vi "Write Switch Setting.vi"(8 "error in (no error)":errorcluster, 10 "Switch Setting":T1, 11 "Switch configuration":refnum<class "Switch configuration.lvclass">) -> (0 "error out":errorcluster, 3 "Switch configuration out":refnum<class "Switch configuration.lvclass">)   [LabVIEW 2025, in "Switch.lvlib" / "Switch configuration.lvclass"]
uses:
  Switch configuration.lvclass
  Switch Instrument Setting.ctl
  Switch configuration.lvclass/Switch configuration.ctl
  <instrlib>/niSwitch/niSwitch.llb/niSwitch Topologies.ctl
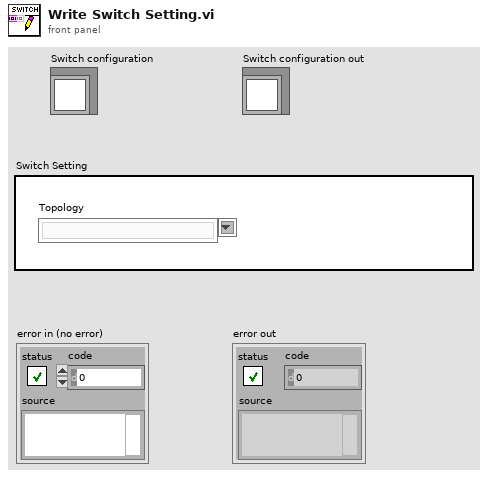
[diagram p1: front panel]
types:
  T1 = typedef "Switch.lvlib/Switch configuration.lvclass/Switch Instrument Setting.ctl" = cluster{"topology name":T2}
  T2 = typedef "niSwitch Topologies.ctl" = string
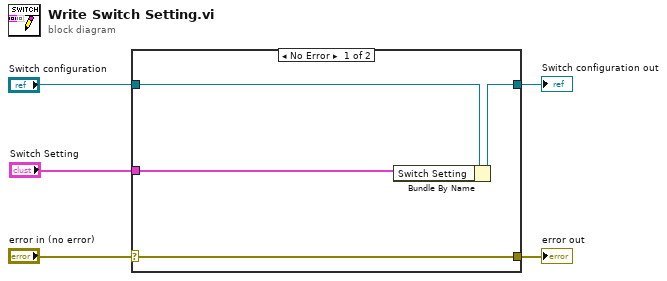
[diagram p0: block diagram]
diagram:
  n1 = case shown="No Error" "error in (no error)" {
    selector: "error in (no error)" -> [w9 w10]
    tunnel: [w9 w10] -> w4
    tunnel: [w7 w11] -> w2
    tunnel: "Switch configuration" -> [w8 w11]
    tunnel: "Switch Setting" -> [w6 _]
    frame No Error {
      n2 = Bundle By Name(cluster=w8, "Switch Setting"=w6) -> (w7:refnum<class "Switch configuration.lvclass">)
    }
    frame Error {
    }
  }
  "error out" <- w4
  "Switch configuration out" <- w2
